vi "Actor Core.vi"(8 "error in":errorcluster, 11 "DIG_IO in":refnum<class "DIG_IO.lvclass">) -> (0 "error out":errorcluster, 3 "Actor out":refnum<class "Actor.lvclass">)   [LabVIEW 2019, in "DIG_IO.lvlib" / "DIG_IO.lvclass"]
doc: "The instrument actor core is only here to distribute panel resolution settings to children classes."
uses:
  Library/DIG_IO.lvclass
  Custom Controls/Single_Bank.ctl
  builds/Engine/Actor Framework.lvlibp/1abvi3w/vi.lib/ActorFramework/Actor/Actor.lvclass
  DIG_IO Messages/Pulse Output Msg/Pulse Output Msg.lvclass/Pulse Output Msg.ctl
  DIG_IO Messages/Toggle IO Enable Msg/Toggle IO Enable Msg.lvclass/Toggle IO Enable Msg.ctl
  DIG_IO Messages/Set by Name Msg/Set by Name Msg.lvclass/Set by Name Msg.ctl
  builds/Engine/Actor Framework.lvlibp/1abvi3w/vi.lib/ActorFramework/Message Enqueuer/Enqueue.vi
  DIG_IO Messages/Pulse Output Msg/Pulse Output Msg.lvclass
  DIG_IO Messages/Toggle IO Enable Msg/Toggle IO Enable Msg.lvclass
  DIG_IO Messages/Clear All Discretes Msg/Clear All Discretes Msg.lvclass
  DIG_IO Messages/Set by Name Msg/Set by Name Msg.lvclass
  DIG_IO Messages/Query Current Msg/Query Current Msg.lvclass
  builds/Instruments/Instruments.lvlibp/Library/Instruments.lvclass
  C:/Users/Public/Documents/Development/builds/Instruments/Instruments.lvlibp/Library/Instruments.lvclass
panel:
  in  "IO_EN":bool
  in  "OpenAll":bool
  in  "Groups":T1(ring)
  in  "Pulse Switch":bool
  in  "Pulse_Period":dbl caption="s"
  in  "Pulse Target":u16(ring) caption="Pulse"
  in  "Active Device":u16(ring)
  out "Tab Control":T2(tab)
  in  "Bank 3":T3
  in  "Bank 2":T3
  in  "Bank 1":T3
  in  "Bank 0":T3
  in  "Bank 7":T3
  in  "Bank 6":T3
  in  "Bank 5":T3
  in  "Bank 4":T3
  in  "Bank 11":T3
  in  "Bank 10":T3
  in  "Bank 9":T3
  in  "Bank 8":T3
  in  "Bank 15":T3
  in  "Bank 14":T3
  in  "Bank 13":T3
  in  "Bank 12":T3
  in  "Bank 19":T3
  in  "Bank 18":T3
  in  "Bank 17":T3
  in  "Bank 16":T3
  in  "Bank 23":T3
  in  "Bank 22":T3
  in  "Bank 21":T3
  in  "Bank 20":T3
  in  "Bank 27":T3
  in  "Bank 26":T3
  in  "Bank 25":T3
  in  "Bank 24":T3
  in  "Bank 31":T3
  in  "Bank 30":T3
  in  "Bank 29":T3
  in  "Bank 28":T3
  in  "Bank 35":T3
  in  "Bank 34":T3
  in  "Bank 33":T3
  in  "Bank 32":T3
  in  "Bank 39":T3
  in  "Bank 38":T3
  in  "Bank 37":T3
  in  "Bank 36":T3
  in  "Bank 43":T3
  in  "Bank 42":T3
  in  "Bank 41":T3
  in  "Bank 40":T3
  in  "Bank 47":T3
  in  "Bank 46":T3
  in  "Bank 45":T3
  in  "Bank 44":T3
  in  "Bank 51":T3
  in  "Bank 50":T3
  in  "Bank 49":T3
  in  "Bank 48":T3
  in  "Bank 55":T3
  in  "Bank 54":T3
  in  "Bank 53":T3
  in  "Bank 52":T3
  in  "Bank 59":T3
  in  "Bank 58":T3
  in  "Bank 57":T3
  in  "Bank 56":T3
  in  "Bank 63":T3
  in  "Bank 62":T3
  in  "Bank 61":T3
  in  "Bank 60":T3
  in  "Bank 67":T3
  in  "Bank 66":T3
  in  "Bank 65":T3
  in  "Bank 64":T3
  in  "Bank 71":T3
  in  "Bank 70":T3
  in  "Bank 69":T3
  in  "Bank 68":T3
  in  "Bank 75":T3
  in  "Bank 74":T3
  in  "Bank 73":T3
  in  "Bank 72":T3
  in  "Bank 79":T3
  in  "Bank 78":T3
  in  "Bank 77":T3
  in  "Bank 76":T3
  in  "Bank 83":T3
  in  "Bank 82":T3
  in  "Bank 81":T3
  in  "Bank 80":T3
  in  "Bank 87":T3
  in  "Bank 86":T3
  in  "Bank 85":T3
  in  "Bank 84":T3
  in  "Bank 91":T3
  in  "Bank 90":T3
  in  "Bank 89":T3
  in  "Bank 88":T3
  in  "Bank 95":T3
  in  "Bank 94":T3
  in  "Bank 93":T3
  in  "Bank 92":T3
  in  "QueryCurrent":bool
  out "Detected Current":dbl
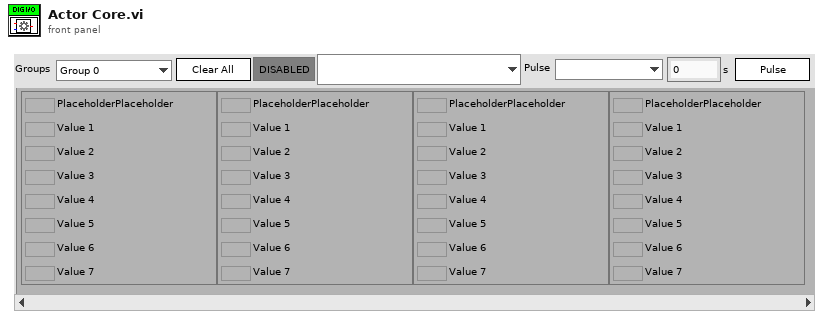
[diagram p1: front panel]
types:
  T1 = enum16{"Group 0", "Group 1", "Group 2", "Group 3", "Group 4", "Group 5", "Group 6", "Group 7", "Group 8", "Group 9", "Group 10", "Group 11", "Group 12", "Group 13", "Group 14", "Group 15", "Group 16", "Group 17", "Group 18", "Group 19", "Group 20", "Group 21", "Group 22", "Group 23", "Housekeeping"}
  T2 = enum32{"Group 0", "Group 1", "Group 2", "Group 3", "Group 4", "Group 5", "Group 6", "Group 7", "Group 8", "Group 9", "Group 10", "Group 11", "Group 12", "Group 13", "Group 14", "Group 15", "Group 16", "Group 17", "Group 18", "Group 19", "Group 20", "Group 21", "Group 22", "Group 23", "Housekeeping"}
  T3 = typedef "DIG_IO.lvlib/DIG_IO.lvclass/Single_Bank.ctl" = cluster{"Value 0":bool, "Value 1":bool, "Value 2":bool, "Value 3":bool, "Value 4":bool, "Value 5":bool, "Value 6":bool, "Value 7":bool}
  T4 = cluster{"Pnl Actor":refnum<event-registration>, "Event Registration Refnum":refnum<event-registration>}
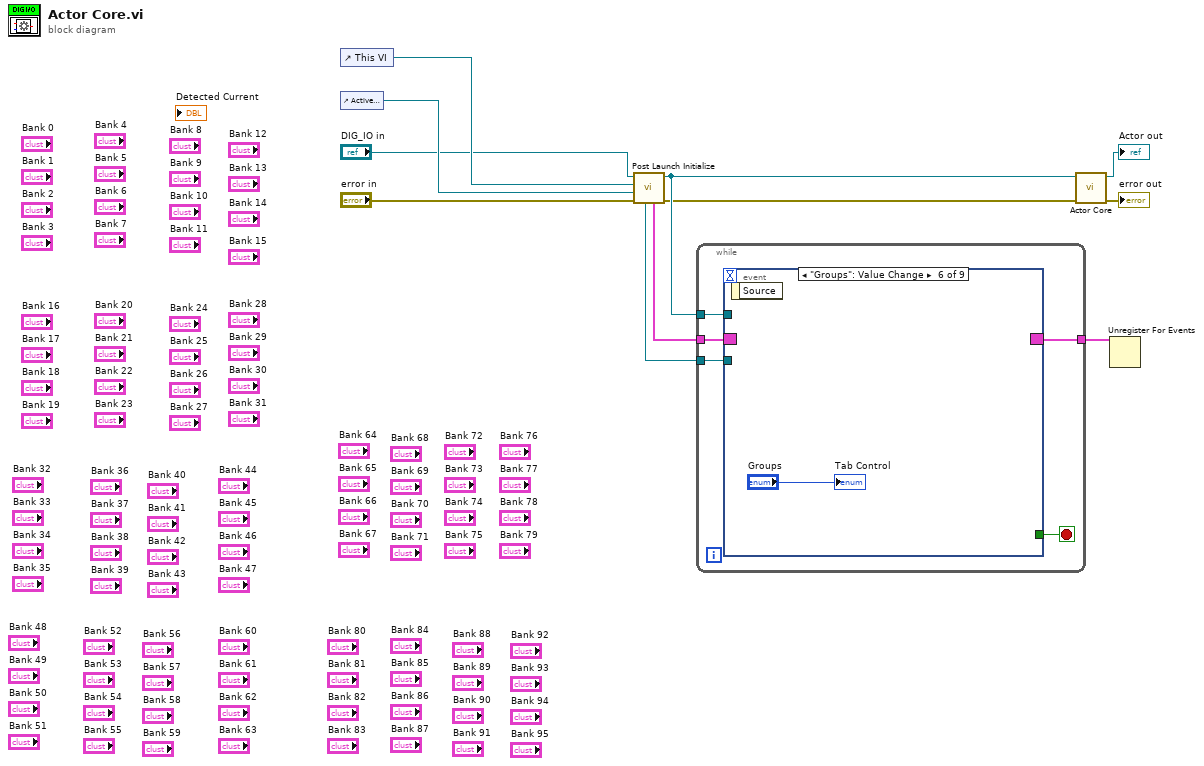
[diagram p0: block diagram]
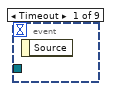
[diagram p2: hidden frame]
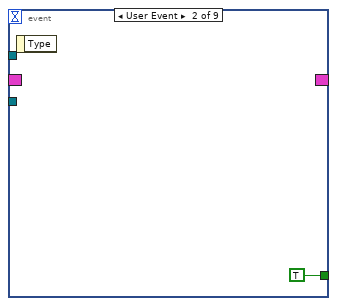
[diagram p3: hidden frame]
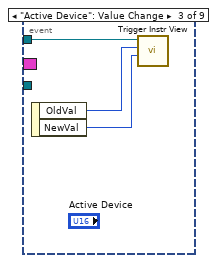
[diagram p4: hidden frame]
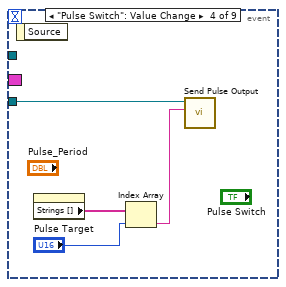
[diagram p5: hidden frame]
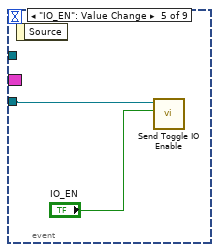
[diagram p6: hidden frame]
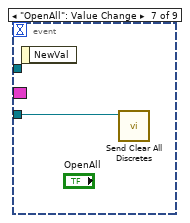
[diagram p7: hidden frame]
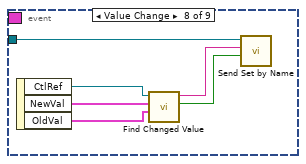
[diagram p8: hidden frame]
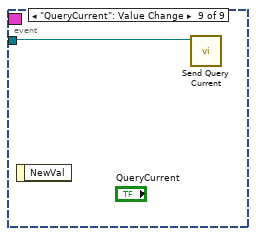
[diagram p9: hidden frame]
diagram:
  n1 = control-ref of="This VI"() -> (w5:refnum<vi>)
  n2 = control-ref of="Active Device"() -> (w4:refnum<vi>)
  n3 = call "Post Launch Initialize.vi"("error in"="error in", "Active Device"=w4, "GUI Reference"=w5, "Instruments in"="DIG_IO in") -> ("error out"=w2:errorcluster, "Instruments out"=w3:refnum<class "DIG_IO.lvclass">, "Registered Events"=w9:T4, "Self Enqueuer"=w8:refnum<class "Message Enqueuer.lvclass">)  [unwired: 4 in]
  n4 = while {
    tunnel: w3 -> [w12]
    tunnel: w9 -> [w16]
    tunnel: w8 -> [w14]
    tunnel: [w15] -> w7
    stop <- w13 stop-if-true
    n5 = event shown="[5] \"Groups\": Value Change" {
      selector: w16 -> [_ _ _ _ _ _ _ _ _]
      dyn-events: [_ _ _ _ _ _ _ _ _] -> w15
      timeout: _ -> [_ _ _ _ _ _ _ _ _]
      tunnel: w14 -> [_ _ _ w22 w26 _ w28 w33 w35]
      tunnel: [_ TRUE _ _ _ _ _ _ _] -> w13
      tunnel: w12 -> [_ _ w20 _ _ _ _ _ _]
      event Timeout {
        n6 = event-data() -> ()  [unwired: 1 in, 1 out]
      }
      event User Event {
        n7 = event-data() -> ()  [unwired: 1 in, 1 out]
      }
      event "Active Device": Value Change {
        n8 = event-data() -> ("OldVal"=w19:u16, "NewVal"=w18:u16)  [unwired: 1 in]
        n9 = call "Trigger Instr View.vi"("New Value"=w18, "Old Value"=w19, "Instruments in"=w20) -> ()  [unwired: 7 in, 2 out]
      }
      event "Pulse Switch": Value Change {
        n10 = event-data() -> ()  [unwired: 1 in, 1 out]
        n11 = property on="Pulse Target" class="Ring (strict)"() -> ("Strings []"=w24:string[])  [unwired: 2 in, 2 out]
        n12 = Index Array(array=w24, index="Pulse Target") -> (element=w21:string)
        n13 = call "Send Pulse Output.vi"("Target"=w21, "Message Enqueuer"=w22) -> ()  [unwired: 8 in, 2 out]
      }
      event "IO_EN": Value Change {
        n14 = event-data() -> ()  [unwired: 1 in, 1 out]
        n15 = call "Send Toggle IO Enable.vi"("IO_EN"="IO_EN", "Message Enqueuer"=w26) -> ()  [unwired: 8 in, 2 out]
      }
      event "Groups": Value Change {
        n16 = event-data() -> ()  [unwired: 1 in, 1 out]
        "Tab Control" <- "Groups"
      }
      event "OpenAll": Value Change {
        n17 = event-data() -> ()  [unwired: 1 in, 1 out]
        n18 = call "Send Clear All Discretes.vi"("Message Enqueuer"=w28) -> ()  [unwired: 9 in, 2 out]
      }
      event Value Change {
        n19 = event-data() -> ("CtlRef"=w34:refnum<vi>, "NewVal"=w30:T3, "OldVal"=w29:T3)  [unwired: 1 in]
        n20 = call "Find Changed Value.vi"("Old Value"=w29, "New Value"=w30, "CtlRef"=w34) -> ("Value"=w31:bool, "Target"=w32:string)  [unwired: 7 in]
        n21 = call "Send Set by Name.vi"("Value"=w31, "Channel Name"=w32, "Message Enqueuer"=w33) -> ()  [unwired: 7 in, 2 out]
      }
      event "QueryCurrent": Value Change {
        n22 = event-data() -> ()  [unwired: 1 in, 1 out]
        n23 = call "Send Query Current.vi"("Message Enqueuer"=w35) -> ()  [unwired: 9 in, 2 out]
      }
    }
  }
  n24 = call-parent "Actor Core.vi"("error in"=w2, "Instruments in"=w3) -> ("error out"=→"error out":errorcluster, "Actor out"=→"Actor out":refnum<class "Actor.lvclass">)  [unwired: 8 in]
  n25 = Unregister For Events(event registration refnum=w7) -> ()  [unwired: 1 in, 1 out]
